vi "Graph Temperature and Setpoint.vi"() -> ()   [LabVIEW 2012]
panel:
  out "Waveform Chart":cluster{dbl, dbl}(graph)
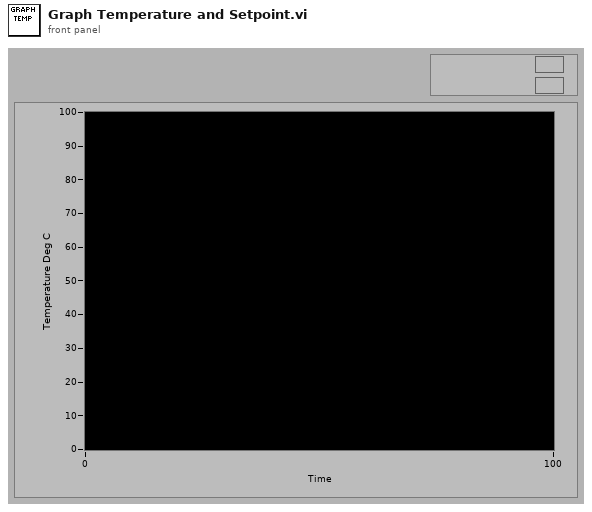
[diagram p1: front panel]
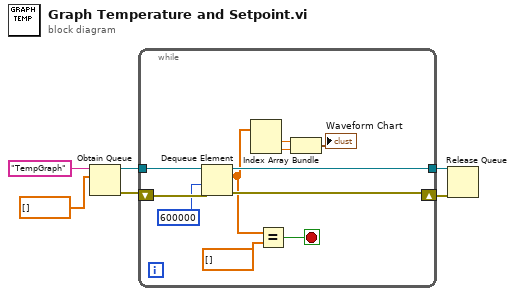
[diagram p0: block diagram]
diagram:
  n1 = Obtain Queue(name (unnamed)="TempGraph", element data type=dbl[] []) -> (queue out=w6:refnum<queue>, error out=w5:errorcluster)  [unwired: 3 in, 1 out]
  n2 = while {
    tunnel: w6 -> [w17]
    shift-right: [w14] -> w1
    shift-left: w5 -> [w16]
    tunnel: [w15] -> w2
    stop <- w12 stop-if-true
    n3 = Dequeue Element(queue=w17, timeout in ms (-1)=600000, error in (no error)=w16) -> (queue out=w15:refnum<queue>, element=w10:dbl[], error out=w14:errorcluster)  [unwired: 1 out]
    n4 = Index Array(array=w10) -> (element #1=w9:dbl, element #2=w8:dbl)  [unwired: 2 in]
    n5 = Equal?(x=w10, y=dbl[] []) -> (x = y?=w12:bool)
    n6 = Bundle(w9, w8) -> (→"Waveform Chart":cluster{dbl, dbl})  [unwired: 1 out]
  }
  n7 = Release Queue(queue=w2, error in (no error)=w1) -> ()  [unwired: 4 out]
